vi "Join Bank DIO.vi"(0 "IN 7:4":fxp<+,4,4>, 1 "IN 3:2":fxp<+,2,2>, 2 "IN 1:0":fxp<+,2,2>, 5 "IN 9:8":fxp<+,2,2>, 7 "IN 11:10":fxp<+,2,2>, 9 "IN 13:12":fxp<+,2,2>, 11 "IN 15:14":fxp<+,2,2>, 12 "IN 17:16":fxp<+,2,2>, 13 "IN 19:18":fxp<+,2,2>) -> (4 "OUT 19:0":fxp<+,20,20> format="%.0b")   [LabVIEW 2021]
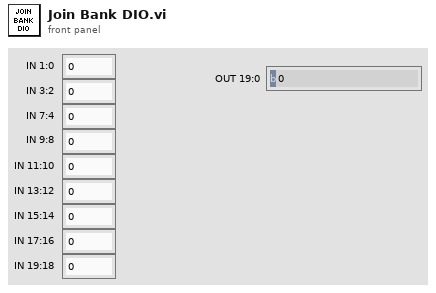
[diagram p1: front panel]
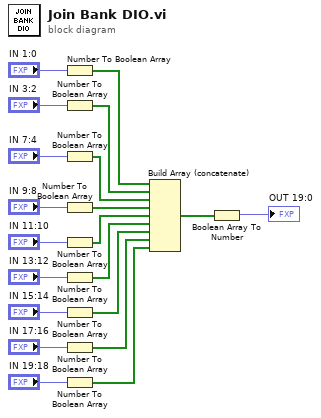
[diagram p0: block diagram]
diagram:
  n1 = Number To Boolean Array(number="IN 1:0") -> (Boolean array=w11:bool[])
  n2 = Number To Boolean Array(number="IN 3:2") -> (Boolean array=w10:bool[])
  n3 = Number To Boolean Array(number="IN 7:4") -> (Boolean array=w9:bool[])
  n4 = Number To Boolean Array(number="IN 9:8") -> (Boolean array=w8:bool[])
  n5 = Number To Boolean Array(number="IN 11:10") -> (Boolean array=w7:bool[])
  n6 = Number To Boolean Array(number="IN 13:12") -> (Boolean array=w6:bool[])
  n7 = Number To Boolean Array(number="IN 15:14") -> (Boolean array=w5:bool[])
  n8 = Number To Boolean Array(number="IN 17:16") -> (Boolean array=w4:bool[])
  n9 = Number To Boolean Array(number="IN 19:18") -> (Boolean array=w3:bool[])
  n10 = Build Array (concatenate)(w11, w10, w9, w8, w7, w6, w5, w4, w3) -> (w2:bool[])
  n11 = Boolean Array To Number(Boolean array=w2) -> (number=→"OUT 19:0":fxp<+,20,20>)
